vi "Execute.vi"(7 "Actor in":refnum<class "Actor.lvclass">, 8 "Error in":errorcluster, 11 "Start Msg in":refnum<class "Start Msg.lvclass">) -> (0 "Error out":errorcluster, 2 "Msg Output":refnum<class "Msg Output.lvclass">, 5 "Actor out":refnum<class "Actor.lvclass">)   [LabVIEW 2020, in "jettl.lvlib" / "Start jettl Msg.lvlib" / "Start Msg.lvlib" / "Start Msg.lvclass"]
doc: "jettl 6.14.1.98\nNathan Davis - Nathan Davis\nCopyright (c) 2026, Nathan Davis\nMIT"
uses:
  Start Msg.lvclass
  Actor/Actor.lvclass
  Msg Output/Msg Output.lvclass
  Start jettl Msg/Start jettl Msg.lvclass
  Start Msg.lvclass/Start Msg.ctl
  Start Msg Output/Start Msg Output.lvlib
  Start Msg Input/Start Msg Input.lvlib
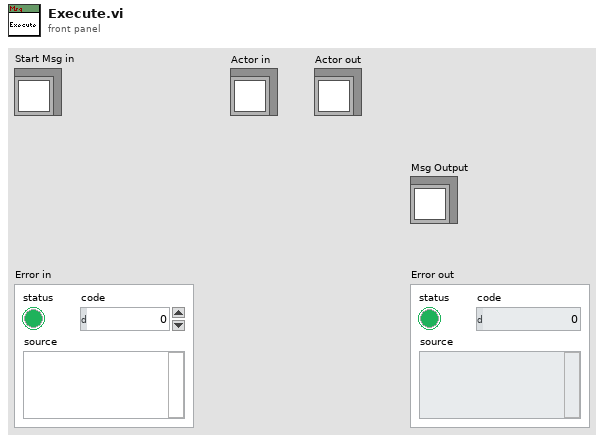
[diagram p1: front panel]
types:
  T1 = typedef "jettl.lvlib/Teller.ctl" = cluster{"Priority":bool, "Time":timestamp, "UID":i32, "Alias":string, "Valid Relation":bool, "Relation":T2, "Called From Msg Library":bool, "Teller Metadata":refnum<class "Teller Metadata.lvclass">}
  T2 = typedef "jettl.lvlib/Relation.ctl" = enum16{"Self", "Parent", "Child"}
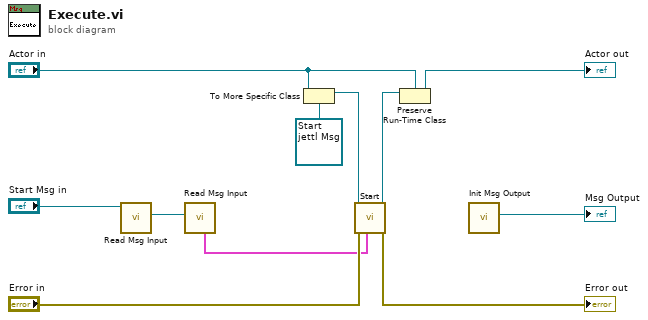
[diagram p0: block diagram]
diagram:
  n1 = call-dynamic "Read Msg Input.vi"("Start Msg in"="Start Msg in") -> ("Msg Input"=w3:refnum<class "Msg Input.lvclass">)  [unwired: 10 in]
  n2 = call "Read Msg Input.vi"("Msg Input"=w3) -> ("Teller"=w1:T1)  [unwired: 10 in]
  n3 = To More Specific Class(target class=refnum<class "Start jettl Msg.lvclass"> refnum ("jettl Msg Template"), reference="Actor in") -> (specific class reference=w10:refnum<class "Start jettl Msg.lvclass">)  [unwired: 1 in, 1 out]
  n4 = call-dynamic "Start.vi"("Teller"=w1, "Error in"="Error in", "Start jettl Msg in"=w10) -> ("Error out"=→"Error out":errorcluster, "Start jettl Msg out"=w9:refnum<class "Start jettl Msg.lvclass">)  [unwired: 7 in]
  n5 = Preserve Run-Time Class(object in=w9, 2:"Actor in") -> (object out=→"Actor out":refnum<class "Actor.lvclass">)  [unwired: 1 in, 1 out]
  n6 = call "Init Msg Output.vi"() -> ("Msg Output"=→"Msg Output":refnum<class "Msg Output.lvclass">)  [unwired: 11 in]
